vi "Init2DAQ.vi"(6 "channel parms":T2={"input impedance"=0, "maximum input frequency"=0.0, "vertical coupling"=1, "probe attenuation"=1.0, "vertical range"=10.0, "vertical offset"=0.0, "channel enabled"=TRUE} {"input impedance" items=["1 mega ohm"=0, "50 ohms"=2]; "vertical coupling" items=["AC", "DC", "Ground"]}, 8 "error in":errorcluster, 9 "reference position":dbl=50.0, 10 "min sample rate":dbl=100000000.0, 11 "resource names":T4={"resource 1"="PXI1Slot2", "resource 2"="PXI1Slot2"}) -> (0 "error out":errorcluster, 3 "instrument out":T3)   [LabVIEW 2013]
uses:
  <instrlib>/niScope/Controls/niScope vertical coupling.ctl
  <instrlib>/niScope/Controls/niScope trigger source digital.ctl
  <instrlib>/niScope/Controls/niScope clock sync pulse source.ctl
  <instrlib>/niScope/Controls/niScope exportable signals.ctl
  <instrlib>/niScope/Controls/niScope export destinations.ctl
  <instrlib>/niScope/Configure/Trigger/niScope Configure Trigger Digital.vi
  <instrlib>/niScope/Configure/Trigger/niScope Configure Trigger Immediate.vi
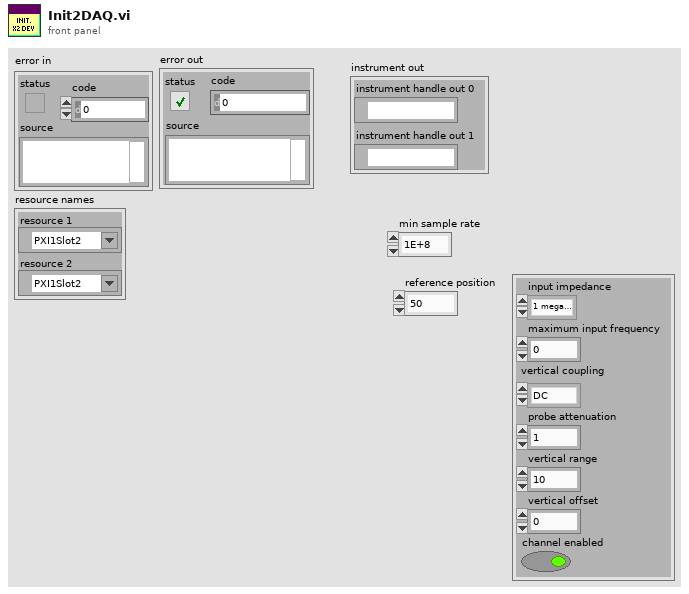
[diagram p1: front panel]
types:
  T1 = typedef "niScope vertical coupling.ctl" = i32
  T2 = cluster{"input impedance":u32, "maximum input frequency":dbl, "vertical coupling":T1, "probe attenuation":dbl, "vertical range":dbl, "vertical offset":dbl, "channel enabled":bool}
  T3 = cluster{"instrument handle out 0":refnum<k15>, "instrument handle out 1":refnum<k15>}
  T4 = cluster{"resource 1":refnum<k15>, "resource 2":refnum<k15>}
  T5 = typedef "niScope export destinations.ctl" = string
  T6 = typedef "niScope exportable signals.ctl" = u16
  T7 = typedef "niScope clock sync pulse source.ctl" = u16
  T8 = typedef "niScope trigger source digital.ctl" = string
  T9 = cluster{"instrument handle out":refnum<k15>, "instrument handle out":refnum<k15>}
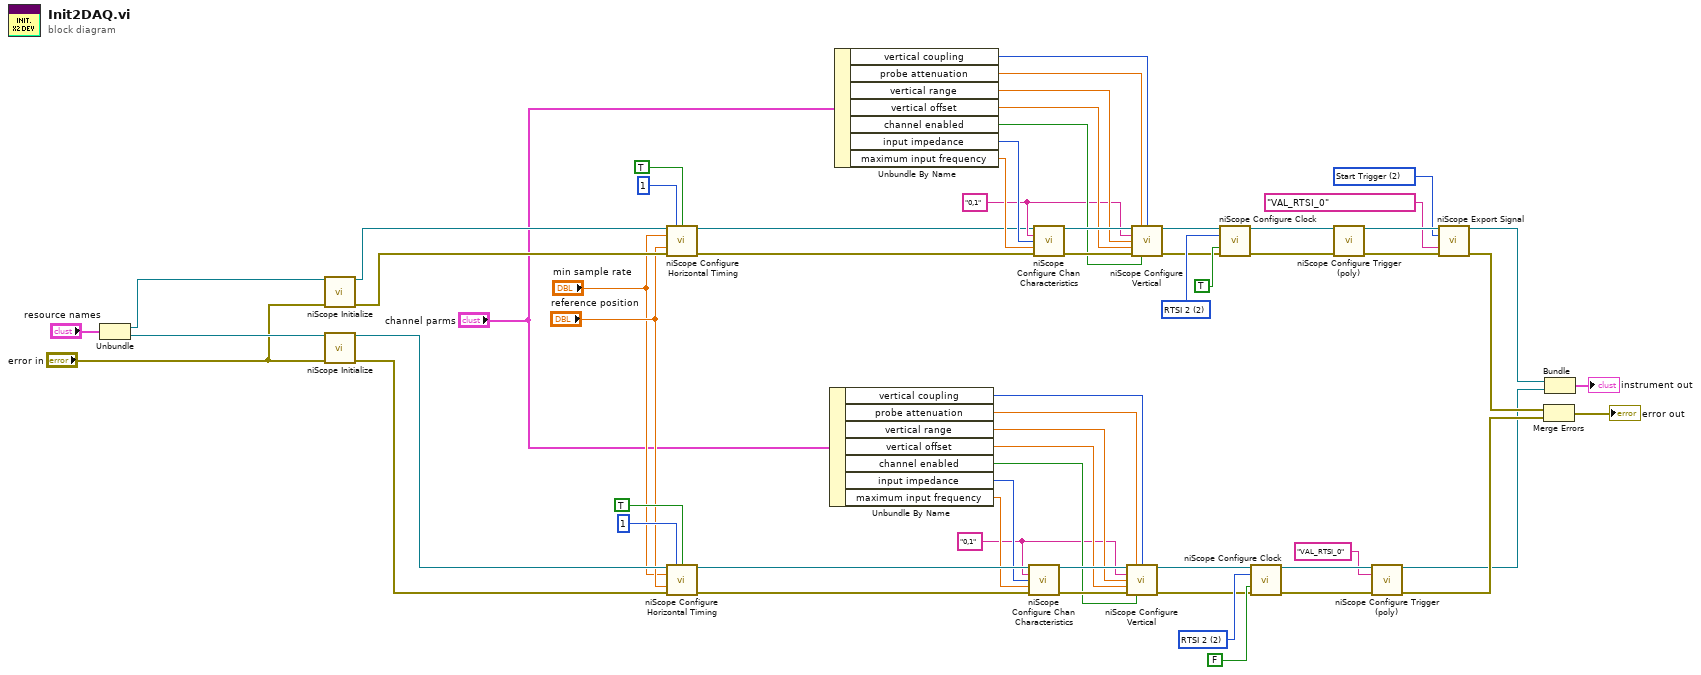
[diagram p0: block diagram]
diagram:
  w6 = "0,1" ("channels")
  w16 = "0,1" ("channels")
  w38 = T6 2 items=["None"=0, "Start Trigger"=2, "Advance Trigger"=5, "Reference Trigger"=1, "End of Record Event"=4, "End of Acquisition Event"=3, "Ready for Start Event"=7, "Ready for Advance Event"=6, "Ready for Reference Event"=10, "Reference Clock"=100, "Sample Clock"=101, "5 Volt Power"=13] ("signal")
  w41 = T7 2 items=["RTSI 0", "RTSI 1", "RTSI 2", "RTSI 3", "RTSI 4", "RTSI 5", "RTSI 6", "PFI 1", "PFI 2", "Internal"] ("clock sync pulse source")
  w45 = T7 2 items=["RTSI 0", "RTSI 1", "RTSI 2", "RTSI 3", "RTSI 4", "RTSI 5", "RTSI 6", "PFI 1", "PFI 2", "Internal"] ("clock sync pulse source")
  n1 = Unbundle("resource names") -> ("resource 1"=w61:refnum<k15>, "resource 2"=w60:refnum<k15>)
  n2 = call <instrlib>:"niScope Initialize.vi"("resource name"=w61, "error in"="error in") -> ("instrument handle"=w58:refnum<k15>, "error out"=w59:errorcluster)  [unwired: 12 in]
  n3 = call <instrlib>:"niScope Initialize.vi"("resource name"=w60, "error in"="error in") -> ("instrument handle"=w55:refnum<k15>, "error out"=w54:errorcluster)  [unwired: 12 in]
  n4 = call <instrlib>:"niScope Configure Horizontal Timing.vi"("instrument handle"=w58, "number of records"=1, "enforce realtime"=TRUE, "min sample rate"="min sample rate", "reference position"="reference position", "error in"=w59) -> ("instrument handle out"=w4:refnum<k15>, "error out"=w3:errorcluster)  [unwired: 1 in, 7 out]
  n5 = call <instrlib>:"niScope Configure Horizontal Timing.vi"("instrument handle"=w55, "number of records"=1, "enforce realtime"=TRUE, "min sample rate"="min sample rate", "reference position"="reference position", "error in"=w54) -> ("instrument handle out"=w29:refnum<k15>, "error out"=w28:errorcluster)  [unwired: 1 in, 7 out]
  n6 = Unbundle By Name("channel parms") -> ("vertical coupling"=w23:T1, "probe attenuation"=w22:dbl, "vertical range"=w21:dbl, "vertical offset"=w20:dbl, "channel enabled"=w19:bool, "input impedance"=w18:u32, "maximum input frequency"=w17:dbl)
  n7 = Unbundle By Name("channel parms") -> ("vertical coupling"=w13:T1, "probe attenuation"=w12:dbl, "vertical range"=w11:dbl, "vertical offset"=w10:dbl, "channel enabled"=w9:bool, "input impedance"=w8:u32, "maximum input frequency"=w7:dbl)
  n8 = call <instrlib>:"niScope Configure Chan Characteristics.vi"("instrument handle"=w29, "channels"=w16, "input impedance"=w18, "maximum input frequency"=w17, "error in"=w28) -> ("instrument handle out"=w27:refnum<k15>, "error out"=w26:errorcluster)  [unwired: 9 out]
  n9 = call <instrlib>:"niScope Configure Chan Characteristics.vi"("instrument handle"=w4, "channels"=w6, "input impedance"=w8, "maximum input frequency"=w7, "error in"=w3) -> ("instrument handle out"=w15:refnum<k15>, "error out"=w14:errorcluster)  [unwired: 9 out]
  n10 = call <instrlib>:"niScope Configure Vertical.vi"("instrument handle"=w27, "probe attenuation"=w22, "vertical coupling"=w23, "channels"=w16, "vertical range"=w21, "vertical offset"=w20, "error in"=w26, "channel enabled"=w19) -> ("instrument handle out"=w24:refnum<k15>, "error out"=w25:errorcluster)  [unwired: 6 out]
  n11 = call <instrlib>:"niScope Configure Vertical.vi"("instrument handle"=w15, "probe attenuation"=w12, "vertical coupling"=w13, "channels"=w6, "vertical range"=w11, "vertical offset"=w10, "error in"=w14, "channel enabled"=w9) -> ("instrument handle out"=w2:refnum<k15>, "error out"=w1:errorcluster)  [unwired: 6 out]
  n12 = call <instrlib>:"niScope Configure Clock.vi"("instrument handle"=w2, "clock sync pulse source"=w41, "master enabled"=TRUE, "error in"=w1) -> ("instrument handle out"=w43:refnum<k15>, "error out"=w42:errorcluster)  [unwired: 10 in]
  n13 = call <instrlib>:"niScope Configure Clock.vi"("instrument handle"=w24, "clock sync pulse source"=w45, "master enabled"=FALSE, "error in"=w25) -> ("instrument handle out"=w47:refnum<k15>, "error out"=w48:errorcluster)  [unwired: 10 in]
  n14 = call-poly <instrlib>:"niScope Configure Trigger (poly).vi"("instrument handle"=w43, "error in"=w42) -> ("instrument handle out"=w40:refnum<k15>, "error out"=w39:errorcluster)  [unwired: 1 in, 11 out]
  n15 = call-poly <instrlib>:"niScope Configure Trigger (poly).vi"("instrument handle"=w47, "trigger source"=T8 "VAL_RTSI_0", "error in"=w48) -> ("instrument handle out"=w30:refnum<k15>, "error out"=w35:errorcluster)  [unwired: 3 in, 8 out]
  n16 = call <instrlib>:"niScope Export Signal.vi"("instrument handle"=w40, "signal"=w38, "output terminal"=T5 "VAL_RTSI_0", "error in"=w39) -> ("instrument handle out"=w31:refnum<k15>, "error out"=w34:errorcluster)  [unwired: 10 in]
  n17 = Merge Errors(w34, w35) -> (→"error out":errorcluster)
  n18 = Bundle("instrument handle out"=w31, "instrument handle out"=w30) -> (→"instrument out":T9)  [unwired: 1 in]
